vi "Delta Between Signals.vi"(4 "second signal":bool, 5 "first signal":bool) -> (1 "delta between signals":u16)   [LabVIEW 2014, in "ni579x Synchronization v2 FPGA.lvlib"]
doc: "Count the number of clock cycles between the first and second signal. When the first signal goes high, begin counting. When the second signal goes high, enable the output feedback node and reset the count on the next cycle."
uses:
  <instrlib>/ni579x/Synchronization/v2/FPGA/ni579x Synchronization v2 FPGA.lvlib
  <instrlib>/_niInstr/Basic Elements/v1/FPGA/niInstr Basic Elements v1 FPGA.lvlib
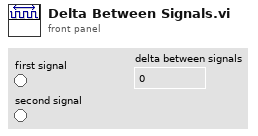
[diagram p1: front panel]
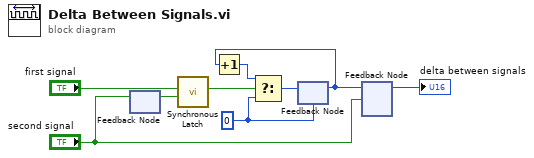
[diagram p0: block diagram]
diagram:
  w4 = u16 0
  n1 = feedback #1() -> (w7:bool)  [unwired: 1 in]
  n2 = feedback-in #1("second signal") -> ()
  n3 = call <instrlib>:"Synchronous Latch.vi"("clear"=w7, "set"="first signal") -> ("out"=w5:bool)  [unwired: 9 in]
  n4 = feedback #2(w4) -> (w2:u16)
  n5 = Increment(x=w2) -> (x+1=w3:u16)
  n6 = Select(t=w3, s=w5, f=w4) -> (s? t:f=w1:u16)
  n7 = feedback-in #2(w1) -> ()
  n8 = feedback #3() -> (→"delta between signals":u16)  [unwired: 1 in]
  n9 = feedback-in #3(w2, "second signal") -> ()
